vi "Array to string converter.vi"(11 "Data In":string[](array[string])) -> (3 "Data Out":string)   [LabVIEW 2021, in "User Interface.lvlib"]
uses:
  User Interface.lvlib
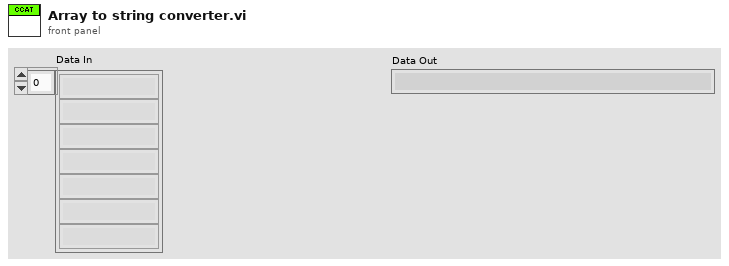
[diagram p1: front panel]
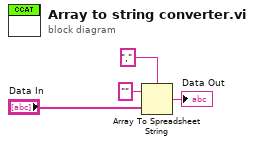
[diagram p0: block diagram]
diagram:
  n1 = Array To Spreadsheet String(delimiter (Tab)=",", array="Data In", 3:"" ("format string")) -> (spreadsheet string=→"Data Out":string)
